vi "Init.vi"(6 "error in":errorcluster, 9 "CaseStructure in":refnum<class "CaseStructure.lvclass">) -> (0 "error out":errorcluster, 3 "CaseStructure out":refnum<class "CaseStructure.lvclass">, 4 "__init__":string)   [LabVIEW 2014, in "CaseStructure.lvclass"]
uses:
  CaseStructure.lvclass
  Python/Parsing/ClassTypeTD.ctl
  Python/Parsing/Python Functions.lvlib
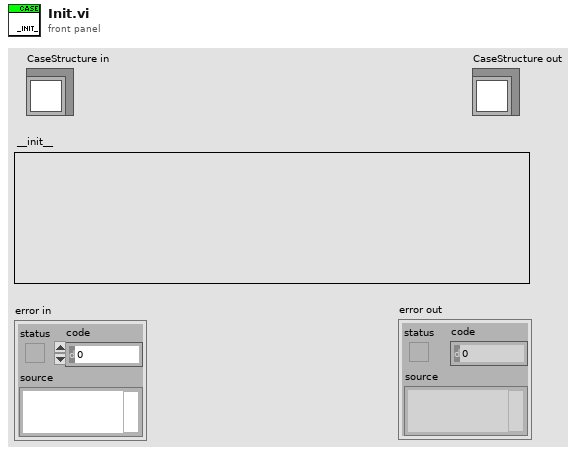
[diagram p1: front panel]
types:
  T1 = typedef "Python Functions.lvlib/ClassTypeTD.ctl" = enum16{"class", "function"}
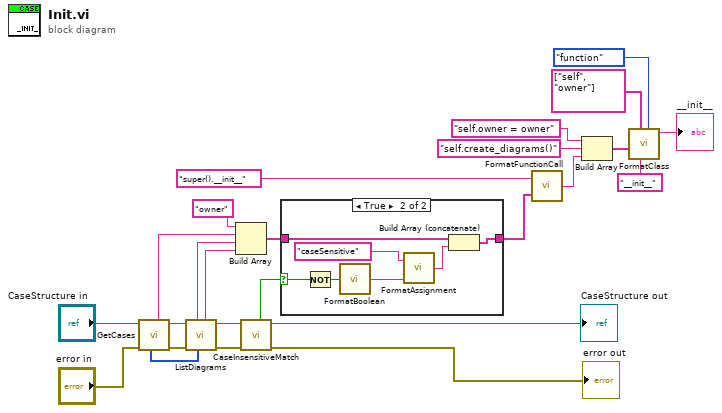
[diagram p0: block diagram]
diagram:
  n1 = call "GetCases.vi"("error in"="error in", "CaseStructure in"="CaseStructure in") -> ("error out"=w20:errorcluster, "CaseStructure out"=w21:refnum<class "CaseStructure.lvclass">, "cases"=w18:string, "diagram indices"=w19:i32[])  [unwired: 4 in]
  n2 = call "ListDiagrams.vi"("diagram indices"=w19, "error in"=w20, "CaseStructure in"=w21) -> ("error out"=w5:errorcluster, "CaseStructure out"=w7:refnum<class "CaseStructure.lvclass">, "default"=w15:string, "diagrams"=w16:string)  [unwired: 5 in]
  n3 = Build Array("owner" ("String"), w18, w16, w15) -> (w2:string[])
  n4 = call "CaseInsensitiveMatch.vi"("error in"=w5, "CaseStructure in"=w7) -> ("error out"=→"error out":errorcluster, "CaseStructure out"=→"CaseStructure out":refnum<class "CaseStructure.lvclass">, "Case Insensitive"=w3:bool)  [unwired: 5 in]
  n5 = case shown="True" w3 {
    selector: w3 -> [_ w29]
    tunnel: w2 -> [w26 w33]
    tunnel: [w26 w32] -> w1
    frame False {
    }
    frame True {
      n6 = Not(x=w29) -> (.not. x?=w27:bool)
      n7 = call "FormatBoolean.vi"("value"=w27) -> ("python object"=w30:string)
      n8 = call "FormatAssignment.vi"("value"=w30, "name"="caseSensitive") -> ("python assignment"=w31:string)
      n9 = Build Array (concatenate)(w33, w31) -> (w32:string[])
    }
  }
  n10 = call "FormatFunctionCall.vi"("parameters"=w1, "function"="super().__init__") -> ("python object"=w10:string)
  n11 = Build Array("self.owner = owner" ("function"), "self.create_diagrams()" ("function"), w10) -> (w9:string[])
  n12 = call "FormatClass.vi"("type"=ClassTypeTD."function", "name"="__init__", "parameters/ancestors"=string[] ["self", "owner"], "body"=w9) -> ("python"=→"__init__":string)  [unwired: 7 in]
